vi "Configure Cascade.vi"(5 "Cascade Mode (0: No Cascade)":u16(ring) items=["No Cascade", "Process Cascade", "Deviation Cascade"], 7 "Unit Address (1)":i16=1, 8 "error in (no error)":errorcluster {"code" format="%.0x"}, 9 "Cascade High Range (19999.0)":dbl=19999.0 format="%.2f", 10 "Cascade Low Range  (-19999.0)":dbl=-19999.0 format="%.2f", 11 "VISA resource name":refnum<visa-resource-name>) -> (0 "error out":errorcluster {"code" format="%.0x"}, 3 "VISA resource name out":refnum<visa-resource-name>)   [LabVIEW 2010]
doc: "This VI configures the cascade mode."
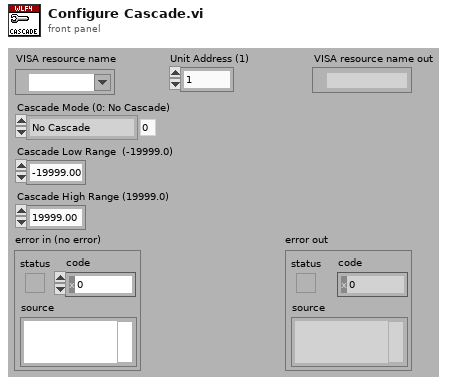
[diagram p1: front panel]
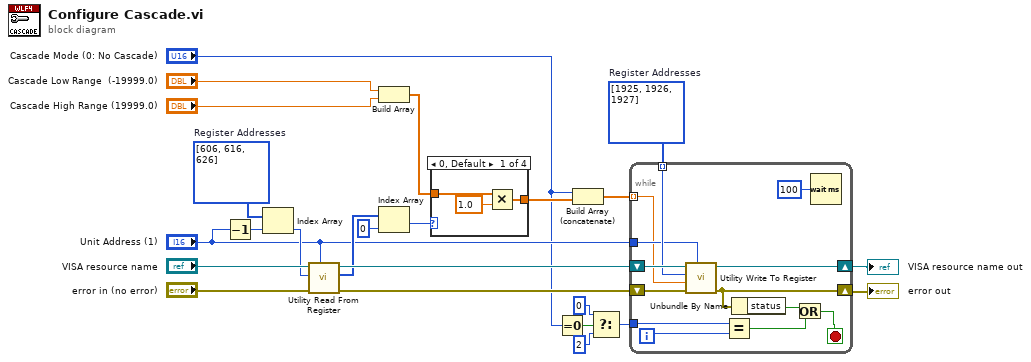
[diagram p0: block diagram]
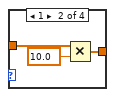
[diagram p2: hidden frame]
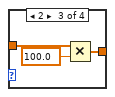
[diagram p3: hidden frame]
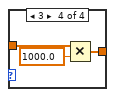
[diagram p4: hidden frame]
diagram:
  w9 = i32[] [606, 616, 626]  # Register Addresses
  w20 = i32[] [1925, 1926, 1927]  # Register Addresses
  n1 = Decrement(x="Unit Address (1)") -> (x-1=w6:i16)
  n2 = Index Array(array=w9, index=w6) -> (element=w8:i32)
  n3 = call "Utility Read From Register.vi"("Unit Address (1)"="Unit Address (1)", "error in (no error)"="error in (no error)", "Register Address (0)"=w8, "VISA resource name"="VISA resource name") -> ("error out"=w15:errorcluster, "Data"=w14:i16[], "VISA resource name out"=w16:refnum<visa-resource-name>)  [unwired: 5 in]
  n4 = Build Array("Cascade Low Range  (-19999.0)", "Cascade High Range (19999.0)") -> (w12:dbl[])
  n5 = Index Array(array=w14, index=0) -> (element=w13:i16)
  n6 = case shown="0, Default" w13 {
    tunnel: [w26 w29 w32 w35] -> w11
    tunnel: w12 -> [w25 w28 w31 w34]
    frame 0, Default {
      n7 = Multiply(x=w25, y=1.0) -> (x*y=w26:dbl[])
    }
    frame 1 {
      n8 = Multiply(x=w28, y=10.0) -> (x*y=w29:dbl[])
    }
    frame 2 {
      n9 = Multiply(x=w31, y=100.0) -> (x*y=w32:dbl[])
    }
    frame 3 {
      n10 = Multiply(x=w34, y=1000.0) -> (x*y=w35:dbl[])
    }
  }
  n11 = Equal To 0?(x="Cascade Mode (0: No Cascade)") -> (x = 0?=w5:bool)
  n12 = Build Array (concatenate)("Cascade Mode (0: No Cascade)", w11) -> (w10:dbl[])
  n13 = Select(t=0, s=w5, f=2) -> (s? t:f=w4:i32)
  n14 = while {
    shift-right: [w47] -> w22
    shift-left: w16 -> [w49]
    shift-right: [w45] -> w21
    shift-left: w15 -> [w48]
    tunnel: w20 -> [w40] mode=indexing
    tunnel: "Unit Address (1)" -> [w39]
    tunnel: w10 -> [w38] mode=indexing
    tunnel: w4 -> [w37]
    i -> [w42]
    stop <- w44 stop-if-true
    n15 = call "Utility Write To Register.vi"("Unit Address (1)"=w39, "error in (no error)"=w48, "Data (0)"=w38, "Register Address (0)"=w40, "VISA resource name"=w49) -> ("error out"=w45:errorcluster, "VISA resource name out"=w47:refnum<visa-resource-name>)  [unwired: 5 in]
    n16 = Equal?(x=w37, y=w42) -> (x = y?=w41:bool)
    n17 = Unbundle By Name(w45) -> ("status"=w43:bool)
    n18 = Or(x=w43, y=w41) -> (x .or. y?=w44:bool)
    n19 = Wait (ms)(milliseconds to wait=u32 100) -> ()  [unwired: 1 out]
  }
  "error out" <- w21
  "VISA resource name out" <- w22
